vi "getSpeed_ShootDualTalonSRX.vi"() -> (0 "Right Speed Ft/SEC":dbl format="%.4f", 3 "Left Speed FT/SEC":dbl format="%.4f")   [LabVIEW 2019, in "ShootDualTalonSRX_Motor_Pair.lvlib"]
uses:
  ShootDualTalonSRX_Motor_Pair.lvlib
  globals_ShootDualTalonSRX.vi
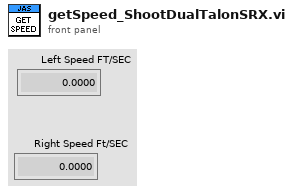
[diagram p1: front panel]
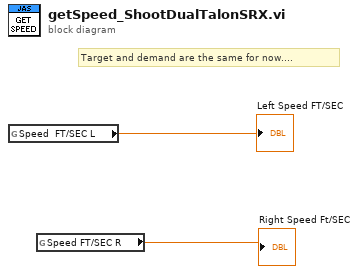
[diagram p0: block diagram]
diagram:
  # "Target and demand are the same for now...."
  n1 = global read "globals_ShootDualTalonSRX.vi" "Speed  FT/SEC L"() -> (→"Left Speed FT/SEC":dbl)
  n2 = global read "globals_ShootDualTalonSRX.vi" "Speed FT/SEC R"() -> (→"Right Speed Ft/SEC":dbl)
